vi "Remove Duplicate Keys.vi"(10 "Variables Value in":string[](array[string]), 11 "Variables Name in":string[](array[string])) -> (1 "Invalid Duplicates":bool, 2 "Variables Value":string[](array[string]), 3 "Variables Name":string[](array[string]))   [LabVIEW 2019]
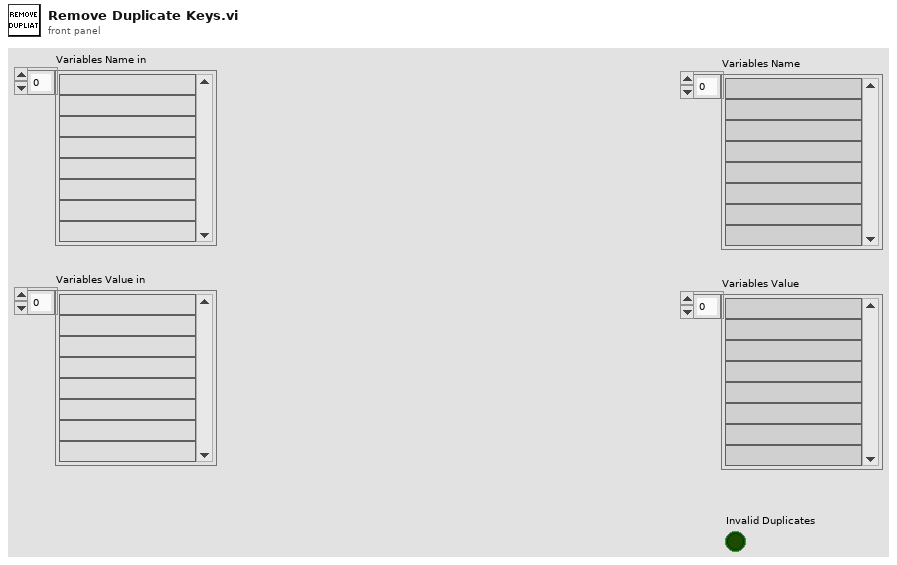
[diagram p1: front panel]
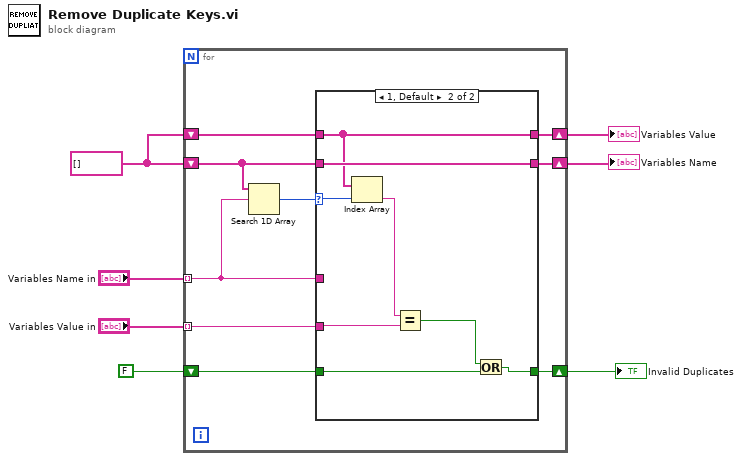
[diagram p0: block diagram]
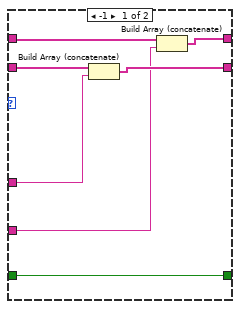
[diagram p2: hidden frame]
diagram:
  w5 = string[] []
  n1 = for {
    tunnel: "Variables Name in" -> [w14] mode=indexing
    tunnel: "Variables Value in" -> [w11] mode=indexing
    shift-right: [w12] -> w3
    shift-left: w5 -> [w15]
    shift-right: [w10] -> w4
    shift-left: w5 -> [w13]
    shift-right: [w9] -> w1
    shift-left: FALSE -> [w8]
    n2 = Search 1D Array(1D array=w15, element=w14) -> (index of element=w16:i32)  [unwired: 1 in]
    n3 = case shown="1, Default" w16 {
      selector: w16 -> [_ w31]
      tunnel: w15 -> [w23 w30]
      tunnel: w14 -> [w22 _]
      tunnel: w13 -> [w20 w29]
      tunnel: [w21 w30] -> w12
      tunnel: w11 -> [w19 w28]
      tunnel: [w18 w29] -> w10
      tunnel: [w17 w26] -> w9
      tunnel: w8 -> [w17 w24]
      frame -1 {
        n4 = Build Array (concatenate)(w23, w22) -> (w21:string[])
        n5 = Build Array (concatenate)(w20, w19) -> (w18:string[])
      }
      frame 1, Default {
        n6 = Index Array(array=w29, index=w31) -> (element=w27:string)
        n7 = Equal?(x=w27, y=w28) -> (x = y?=w25:bool)
        n8 = Or(x=w25, y=w24) -> (x .or. y?=w26:bool)
      }
    }
  }
  "Variables Value" <- w4
  "Variables Name" <- w3
  "Invalid Duplicates" <- w1
